vi "Analys menu.vi"(8 "error in (no error)":errorcluster, 10 "data in":T3 caption="Cluster") -> (0 "error out":errorcluster, 1 "close win?":bool, 2 "data out":T1)   [LabVIEW 2019]
uses:
  TypeDef/Analys type.ctl
  TypeDef/Analys data.ctl
panel:
  in  "Apply":bool
  # "Введите необходимые параметры для анализа"
  # "мм"
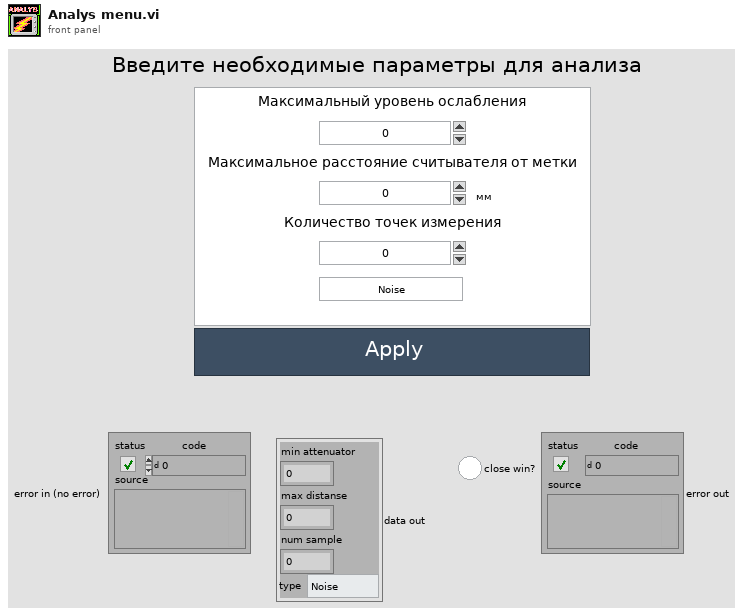
[diagram p1: front panel]
types:
  T1 = typedef "Analys data.ctl" = cluster{"min attenuator":dbl, "max distanse":dbl, "num sample":dbl, "type":T2}
  T2 = typedef "Analys type.ctl" = enum16{"Noise", "Distance"}
  T3 = cluster{"Максимальный уровень ослабления":dbl, "Максимальное расстояние считывателя от метки":dbl, "Количество точек измерения":dbl, "Enum":T2}
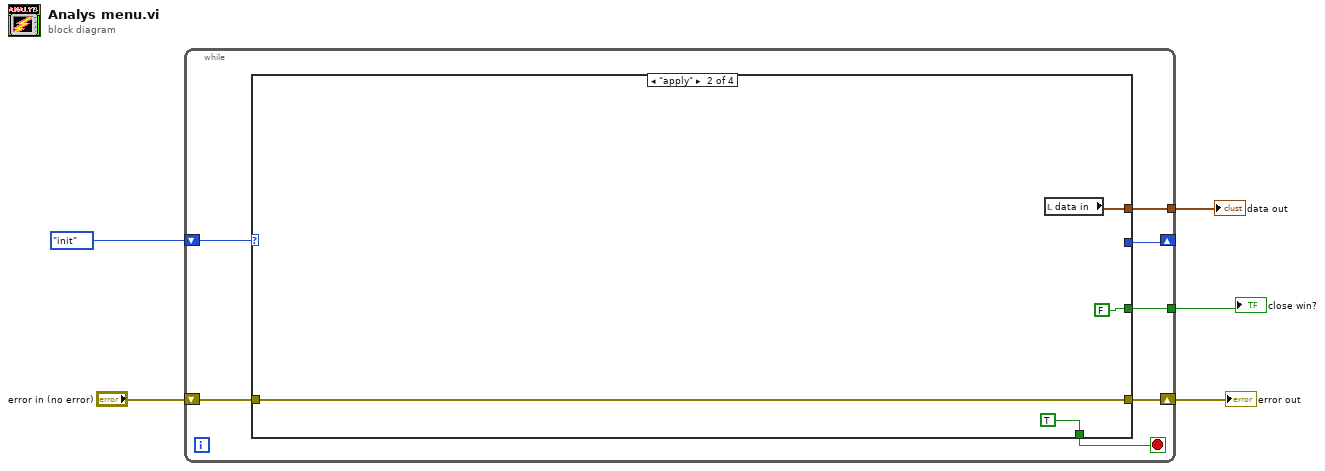
[diagram p0: block diagram]
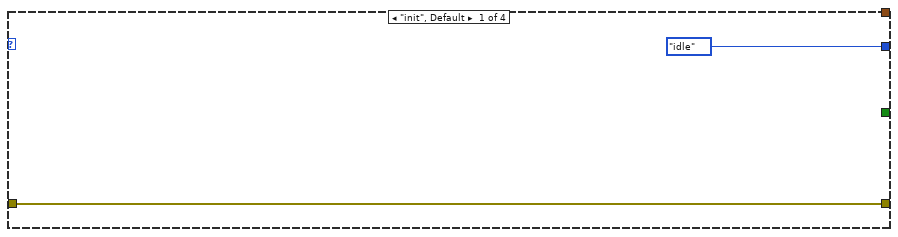
[diagram p2: hidden frame]
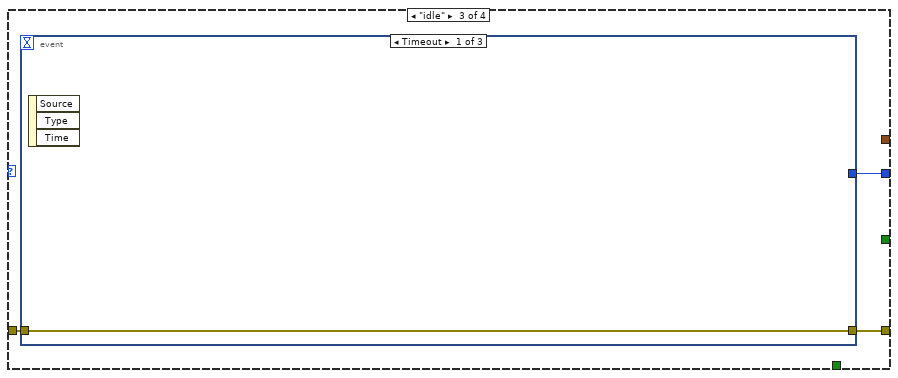
[diagram p3: hidden frame]
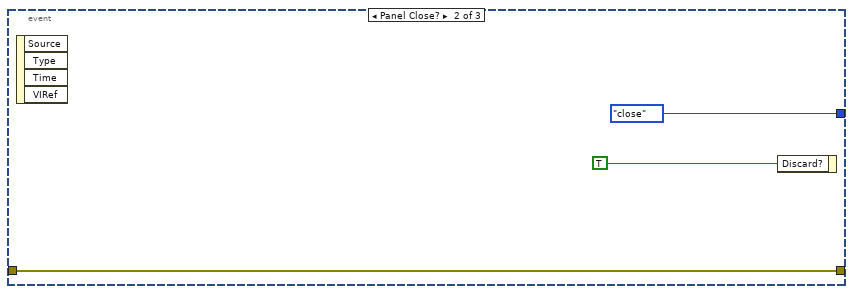
[diagram p4: hidden frame]
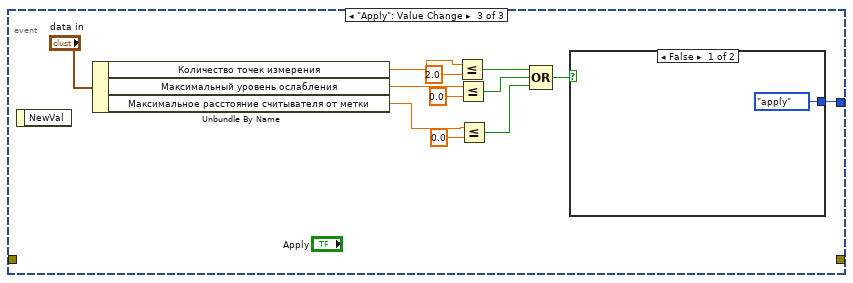
[diagram p5: hidden frame]
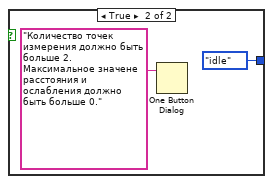
[diagram p6: hidden frame]
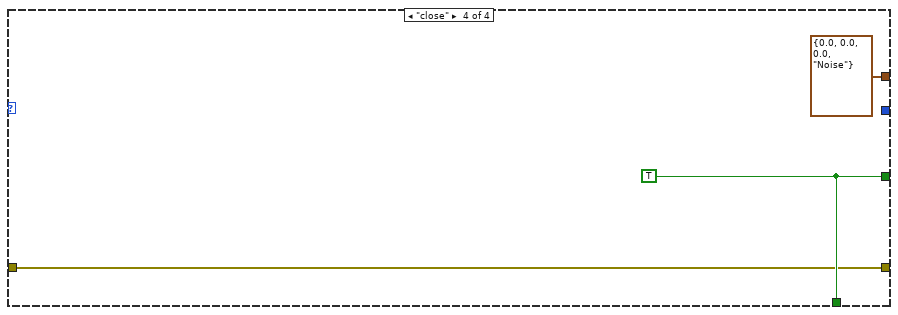
[diagram p7: hidden frame]
diagram:
  n1 = while {
    shift-right: [w11] -> _
    shift-left: enum16{"idle", "init", "close", "apply"}."init" -> [w12]
    tunnel: [w9] -> w4
    shift-right: [w7] -> w2
    shift-left: "error in (no error)" -> [w8]
    tunnel: [w6] -> w1
    stop <- w10 stop-if-true
    n2 = case shown="\"apply\"" w12 {
      tunnel: [enum16{"idle", "init", "close", "apply"}."idle" _ w21 _] -> w11
      tunnel: [_ TRUE _ w43] -> w10
      tunnel: [_ FALSE _ w43] -> w9
      tunnel: w8 -> [w14 w18 w20 w42]
      tunnel: [w14 w18 w19 w42] -> w7
      tunnel: [_ w15 _ T3 {"Максимальный уровень ослабления"=0.0, "Максимальное расстояние считывателя от метки"=0.0, "Количество точек измерения"=0.0, "Enum"=enum."Noise"} ("data in")] -> w6
      frame "init", Default {
      }
      frame "apply" {
        n3 = local read "data in"() -> (w15:T3)
      }
      frame "idle" {
        n4 = event shown="[0] Timeout" {
          selector: _ -> [_ _ _]
          dyn-events: _ -> [_ _ _]
          timeout: _ -> [_ _ _]
          tunnel: [_ enum16{"idle", "init", "close", "apply"}."close" w37] -> w21
          tunnel: w20 -> [w22 w23 _]
          tunnel: [w22 w23 _] -> w19
          event Timeout {
            n5 = event-data() -> ()  [unwired: 1 in, 3 out]
          }
          event Panel Close? {
            n6 = event-data() -> ()  [unwired: 1 in, 4 out]
            n7 = event-data("Discard?"=TRUE) -> ()  [unwired: 1 in, 1 out]
          }
          event "Apply": Value Change {
            n8 = event-data() -> ()  [unwired: 1 in, 1 out]
            n9 = Unbundle By Name("data in") -> ("Количество точек измерения"=w32:dbl, "Максимальный уровень ослабления"=w31:dbl, "Максимальное расстояние считывателя от метки"=w30:dbl)
            n10 = Less Or Equal?(x=w32, y=2.0) -> (x <= y?=w29:bool)
            n11 = Less Or Equal?(x=w31, y=0.0) -> (x <= y?=w28:bool)
            n12 = Less Or Equal?(x=w30, y=0.0) -> (x <= y?=w27:bool)
            n13 = Compound Arithmetic op=OR(w29, w28, w27) -> (w26:bool)
            n14 = case shown="False" w26 {
              tunnel: [enum16{"idle", "init", "close", "apply"}."apply" enum16{"idle", "init", "close", "apply"}."idle"] -> w37
              frame False {
              }
              frame True {
                n15 = One Button Dialog(message="Количество точек измерения должно быть больше 2. Максимальное значене расстояния и ослабления должно быть больше 0.") -> ()  [unwired: 1 in, 1 out]
              }
            }
          }
        }
      }
      frame "close" {
        w43 = TRUE
      }
    }
  }
  "error out" <- w2
  "close win?" <- w4
  "data out" <- w1
